vi "CryoServer Send Piper Passthrough.vi"(8 "error in (no error)":errorcluster, 9 "Piper Command":string, 10 "Piper Board ID (Hex)":u32 format="%x", 11 "CryoServer in":refnum<class "CryoServer.lvclass">) -> (0 "error out":errorcluster, 2 "Response":string, 3 "CryoServer out":refnum<class "CryoServer.lvclass">)   [LabVIEW 2024, in "CryoServer.lvclass"]
uses:
  CryoServer.lvclass
  CryoServer.lvclass/CryoServer.ctl
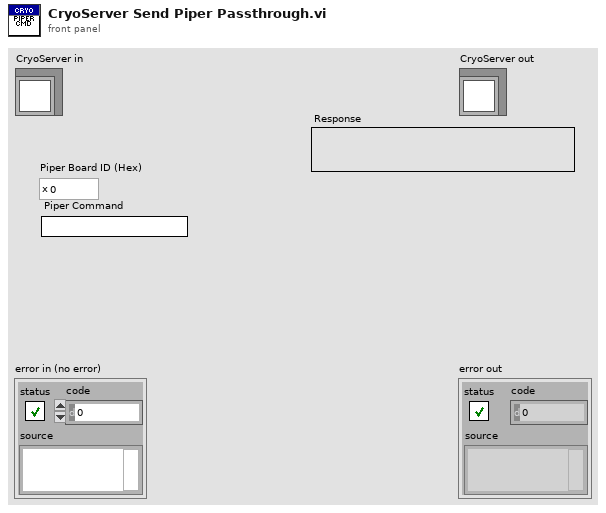
[diagram p1: front panel]
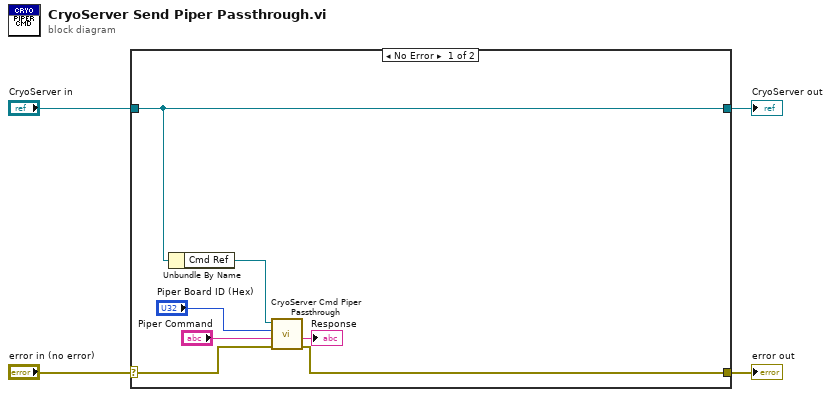
[diagram p0: block diagram]
diagram:
  n1 = case shown="No Error" "error in (no error)" {
    selector: "error in (no error)" -> [w7 w13]
    tunnel: [w6 w13] -> w3
    tunnel: [w11 w12] -> w1
    tunnel: "CryoServer in" -> [w11 w12]
    frame No Error {
      n2 = Unbundle By Name(w11) -> ("Cmd Ref"=w10:refnum<k5>)
      n3 = call "CryoServer Cmd Piper Passthrough.vi"("error in (no error)"=w7, "Piper Command"="Piper Command", "Piper Board ID (Hex)"="Piper Board ID (Hex)", "connection ID"=w10) -> ("error out"=w6:errorcluster, "Response"=→"Response":string)  [unwired: 4 in, 2 out]
    }
    frame Error {
    }
  }
  "error out" <- w3
  "CryoServer out" <- w1
